vi "minimal_fw103h.vi"() -> ()   [LabVIEW 2020]
uses:
  C:/Users/OPMuser/Documents/labview/fw103/Thorlabs.MotionControl.Controls.dll
  Thorlabs.MotionControl.Controls.dll
  C:/Users/OPMuser/Documents/labview/fw103/Thorlabs.MotionControl.Benchtop.StepperMotorCLI.dll
  Thorlabs.MotionControl.Benchtop.StepperMotorCLI.dll
panel:
  in  "stop":bool
  in  "SerialNumber":string="40154488"
  in  "BenchtopStepperControl":refnum<k24>(container)
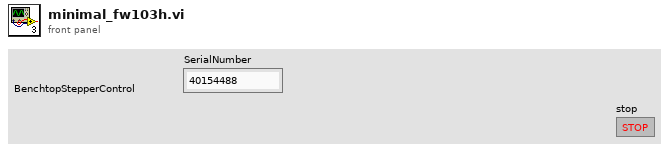
[diagram p1: front panel]
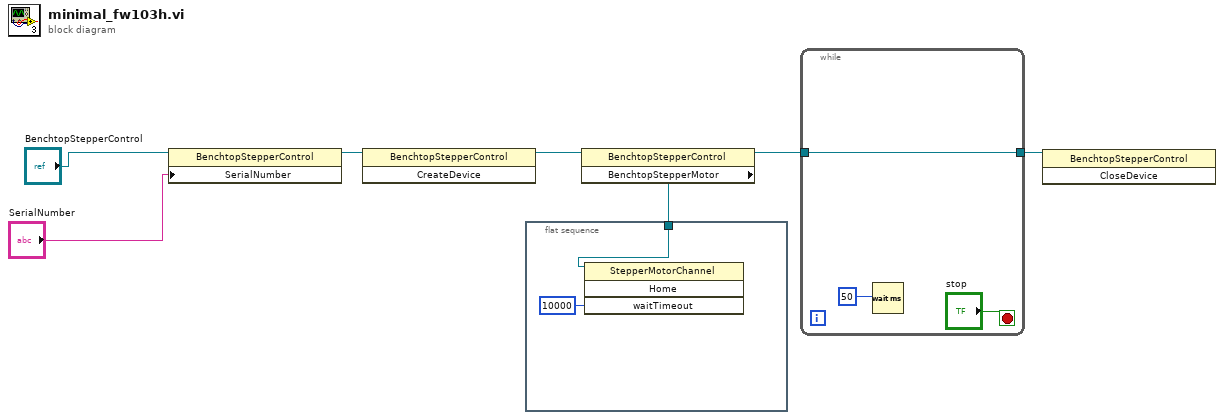
[diagram p0: block diagram]
diagram:
  n1 = property class="BenchtopStepperControl"(reference="BenchtopStepperControl", "SerialNumber"="SerialNumber") -> (reference out=w5:refnum<k24>)  [unwired: 1 in, 1 out]
  n2 = invoke class="BenchtopStepperControl" method="CreateDevice"(reference=w5) -> (reference out=w4:refnum<k24>)  [unwired: 2 in, 2 out]
  n3 = flat-sequence {
    tunnel: w1 -> [w9]
    frame #0 {
      n4 = invoke class="StepperMotorChannel" method="Home"(reference=w9, "waitTimeout"=10000) -> ()  [unwired: 2 in, 4 out]
    }
  }
  n5 = property class="BenchtopStepperControl"(reference=w4) -> (reference out=w3:refnum<k24>, "BenchtopStepperMotor"=w1:refnum<k24>)  [unwired: 1 in, 1 out]
  n6 = while {
    tunnel: w3 -> [w11]
    tunnel: [w11] -> w2
    stop <- "stop" stop-if-true
    n7 = Wait (ms)(milliseconds to wait=u32 50 ("millisecond timer value")) -> ()  [unwired: 1 out]
  }
  n8 = invoke class="BenchtopStepperControl" method="CloseDevice"(reference=w2) -> ()  [unwired: 2 in, 3 out]
